vi "Initialize.vi"(11 "data in":refnum<class "EventMessengerData.lvclass">) -> (1 "Event Registration Refnum":refnum<event-registration>, 3 "data out":refnum<class "EventMessengerData.lvclass">)   [LabVIEW 2019, in "Cmd-Data Event Messenger.lvlib" / "EventMessengerData.lvclass"]
uses:
  EventMessengerData.lvclass
  Event Data.ctl
  EventMessengerData.lvclass/EventMessengerData.ctl
  Cmd-Data Event Messenger.lvlib
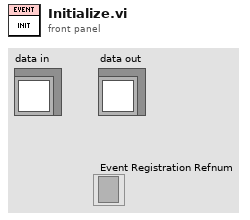
[diagram p1: front panel]
types:
  T1 = typedef "Cmd-Data Event Messenger.lvlib/Event Data.ctl" = cluster{"msg":cluster{"cmd":string, "data":variant}, "valid?":bool, "last?":bool, "aborted?":bool, "priority?":bool}
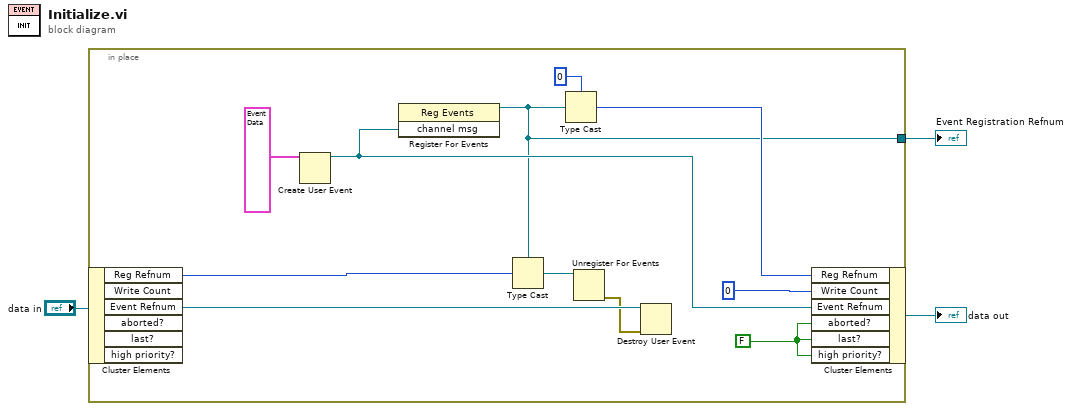
[diagram p0: block diagram]
diagram:
  n1 = in-place {
    in-place-border: [w4] -> w1
    w6 = FALSE ("aborted?")
    n2 = in-place-cluster #1("data in") -> ("Reg Refnum"=w14:u32, "Event Refnum"=w12:refnum<user-event>)  [unwired: 4 out]
    n3 = Create User Event(user event datatype=T1 {"msg"={"cmd"="", "data"=variant}, "valid?"=FALSE, "last?"=FALSE, "aborted?"=FALSE, "priority?"=FALSE} ("channel msg")) -> (user event=w8:refnum<user-event>)  [unwired: 1 in, 1 out]
    n4 = register-events(w8) -> (reference out=w4:refnum<event-registration>)  [unwired: 2 in, 1 out]
    n5 = Type Cast(type=w4, x=w14) -> (*(type *) &x=w13:refnum<event-registration>)
    n6 = Type Cast(type=u32 0 ("Reg Refnum"), x=w4) -> (*(type *) &x=w7:u32)
    n7 = Unregister For Events(event registration refnum=w13) -> (error out=w11:errorcluster)  [unwired: 1 in]
    n8 = Destroy User Event(user event=w12, error in=w11) -> ()  [unwired: 1 out]
    n9 = in-place-cluster #1("Reg Refnum"=w7, "Write Count"=u32 0 ("Registration Count"), "Event Refnum"=w8, "aborted?"=w6, "last?"=w6, "high priority?"=w6) -> (→"data out":refnum<class "EventMessengerData.lvclass">)
  }
  "Event Registration Refnum" <- w1
